vi "Read MODEL.vi"(8 "error in (no error)":errorcluster, 11 "CONTROLLER in":refnum<class "CONTROLLER.lvclass">) -> (0 "error out":errorcluster, 2 "MODEL.lvclass":refnum<class "MODEL.lvclass">, 3 "CONTROLLER out":refnum<class "CONTROLLER.lvclass">)   [LabVIEW 2013, in "CONTROLLER.lvclass"]
uses:
  CONTROLLER.lvclass
  Model/base/MODEL.lvclass
  CONTROLLER.lvclass/CONTROLLER.ctl
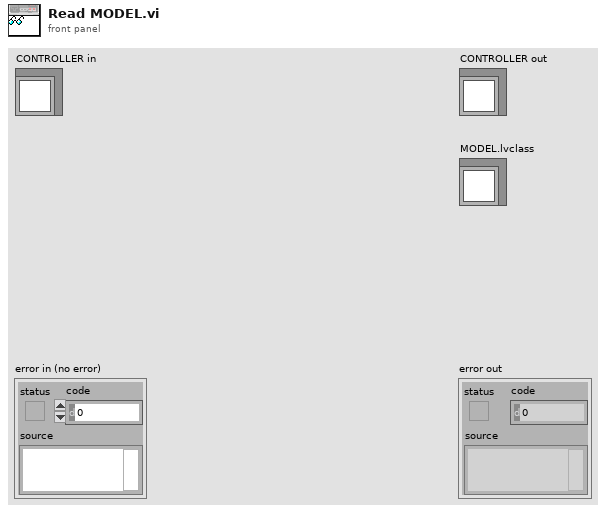
[diagram p1: front panel]
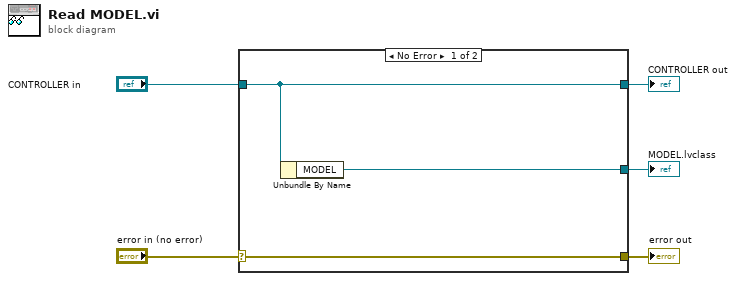
[diagram p0: block diagram]
diagram:
  n1 = case shown="No Error" "error in (no error)" {
    selector: "error in (no error)" -> [w8 w9]
    tunnel: [w8 w9] -> w4
    tunnel: [w7 w10] -> w2
    tunnel: "CONTROLLER in" -> [w7 w10]
    tunnel: [w6 _] -> w1
    frame No Error {
      n2 = Unbundle By Name(w7) -> ("MODEL"=w6:refnum<class "MODEL.lvclass">)
    }
    frame Error {
    }
  }
  "error out" <- w4
  "CONTROLLER out" <- w2
  "MODEL.lvclass" <- w1
